vi "Element Type.vi"(11 "2WayValve in":refnum<class "2WayValve.lvclass">) -> (2 "Control Type":string)   [LabVIEW 2020, in "VolatusGUI.lvlib" / "2WayValve.lvclass"]
uses:
  2WayValve.lvclass
  2WayValve.lvclass/2WayValve.ctl
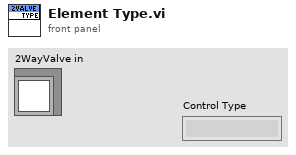
[diagram p1: front panel]
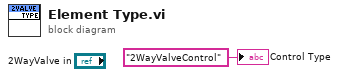
[diagram p0: block diagram]
diagram:
  "Control Type" <- "2WayValveControl" ("Control Type")
